vi "Output CS Refs.vi"(11 "Output CS in":refnum<vi>) -> (2 "Write Frame":refnum<vi>, 3 "Output CS":refnum<vi>, 5 "Close Term":refnum<vi>)   [LabVIEW 2020, in "FlexBlocks.lvlib"]
uses:
  FlexBlocks.lvlib
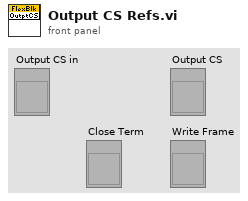
[diagram p1: front panel]
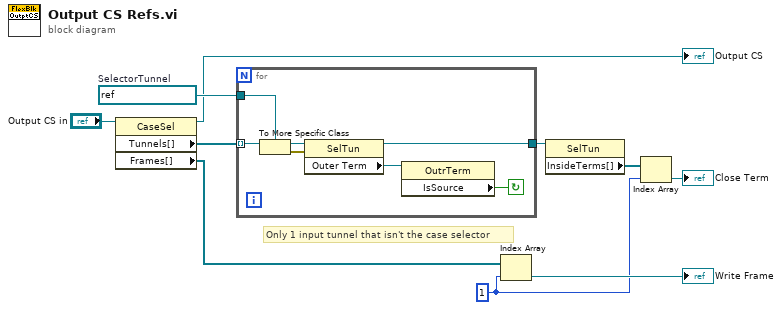
[diagram p0: block diagram]
diagram:
  w2 = 1 ("index")
  w9 = refnum<vi> refnum  # SelectorTunnel
  # "Only 1 input tunnel that isn't the case selector"
  n1 = property class="CaseSel"(reference="Output CS in") -> (reference out=→"Output CS":refnum<vi>, "Tunnels[]"=w10:refnum<vi>[], "Frames[]"=w7:refnum<vi>[])  [unwired: 1 in, 1 out]
  n2 = for {
    tunnel: w10 -> [w17] mode=indexing
    tunnel: w9 -> [w15]
    tunnel: [w12] -> w4
    stop <- w11 continue-if-true
    n3 = To More Specific Class(target class=w15, reference=w17) -> (specific class reference=w16:refnum<vi>, error out=w13:errorcluster)  [unwired: 1 in]
    n4 = property class="SelTun"(reference=w16, error in=w13) -> (reference out=w12:refnum<vi>, "Outer Term"=w14:refnum<vi>)  [unwired: 1 out]
    n5 = property class="OutrTerm"(reference=w14) -> ("IsSource"=w11:bool)  [unwired: 1 in, 2 out]
  }
  n6 = Index Array(array=w7, index=w2) -> (element=→"Write Frame":refnum<vi>)
  n7 = property class="SelTun"(reference=w4) -> ("InsideTerms[]"=w3:refnum<vi>[])  [unwired: 1 in, 2 out]
  n8 = Index Array(array=w3, index=w2) -> (element=→"Close Term":refnum<vi>)
